vi "check RTU validity.vi"(8 "error in (no error)":errorcluster, 10 "unit ID":u8, 11 "unsigned byte array":u8[](array[numeric])) -> (0 "error out":errorcluster, 1 "valid packet":bool, 2 "valid PDU":bool, 3 "Modbus data unit out":refnum<class "Modbus Data Unit (PDU).lvclass">)   [LabVIEW 2020, in "SubVIs.lvlib" / "RTU Data Unit.lvclass"]
uses:
  <vilib>/Modbus/subvis/Transmission Data Unit (ADU)/RTU Data Unit/RTU Data Unit.lvclass
  <vilib>/Modbus/subvis/Modbus Data Unit (PDU)/Modbus Data Unit (PDU).lvclass
  <vilib>/Modbus/subvis/Modbus Data Unit (PDU)/Modbus Data Unit (PDU).lvclass/Modbus Data Unit (PDU).ctl
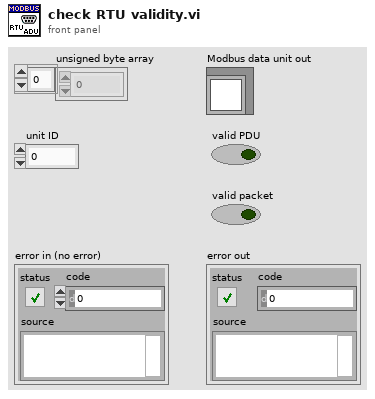
[diagram p1: front panel]
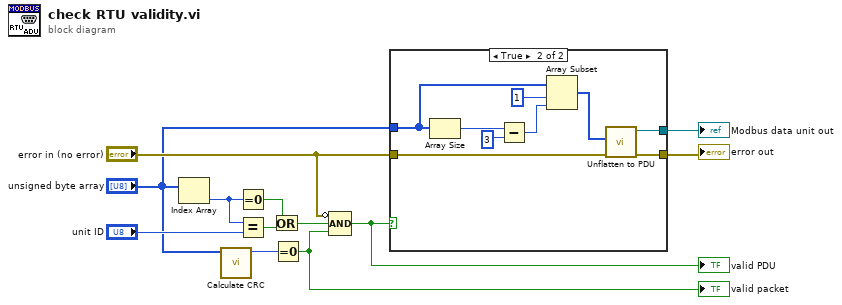
[diagram p0: block diagram]
diagram:
  n1 = Index Array(array="unsigned byte array") -> (element=w6:u8)  [unwired: 1 in]
  n2 = call <vilib>:"Calculate CRC.vi"("data"="unsigned byte array") -> ("CRC-16"=w2:u16)  [unwired: 10 in]
  n3 = Equal To 0?(x=w6) -> (x = 0?=w7:bool)
  n4 = Equal?(x=w6, y="unit ID") -> (x = y?=w8:bool)
  n5 = Or(x=w7, y=w8) -> (x .or. y?=w10:bool)
  n6 = Equal To 0?(x=w2) -> (x = 0?=w5:bool)
  "valid packet" <- w5
  n7 = Compound Arithmetic op=AND(invert "error in (no error)", w10, w5) -> (w4:bool)
  "valid PDU" <- w4
  n8 = case shown="True" w4 {
    tunnel: "error in (no error)" -> [w13 w15]
    tunnel: "unsigned byte array" -> [_ w18]
    tunnel: [w13 w17] -> w12
    tunnel: [_ w14] -> w1
    frame False {
    }
    frame True {
      n9 = Array Size(array=w18) -> (size(s)=w21:i32)
      n10 = Subtract(x=w21, y=3) -> (x-y=w19:i32)
      n11 = Array Subset(array=w18, index=1, length=w19) -> (w16:u8[])
      n12 = call <vilib>:"Unflatten to PDU.vi"("error in (no error)"=w15, "Modbus data unit data"=w16) -> ("error out"=w17:errorcluster, "Modbus data unit out"=w14:refnum<class "Modbus Data Unit (PDU).lvclass">)  [unwired: 8 in]
    }
  }
  "error out" <- w12
  "Modbus data unit out" <- w1
